vi "Write Humidifier T.vi"(8 "error in (no error)":errorcluster, 10 "Humidifier T":cluster{"Hum 1":sgl, "Hum 2":sgl}, 11 "cCRDS Data in":refnum<class "cCRDS Data.lvclass">=refnum) -> (0 "error out":errorcluster, 3 "cCRDS Data out":refnum<class "cCRDS Data.lvclass">)   [LabVIEW 2015, in "cCRDS Data.lvclass"]
uses:
  cCRDS Data.lvclass
  cCRDS Data.lvclass/cCRDS Data.ctl
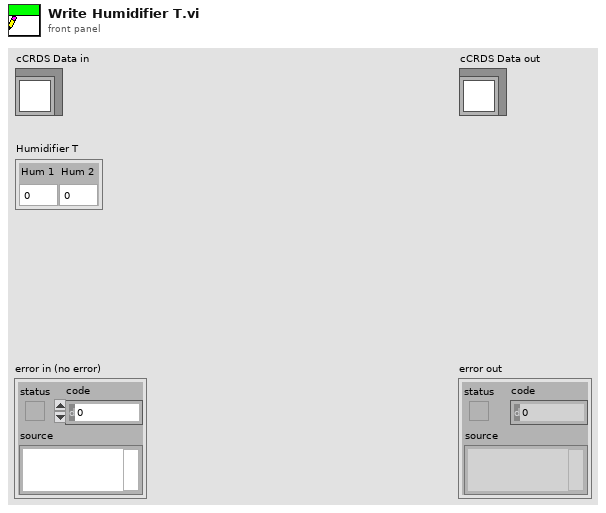
[diagram p1: front panel]
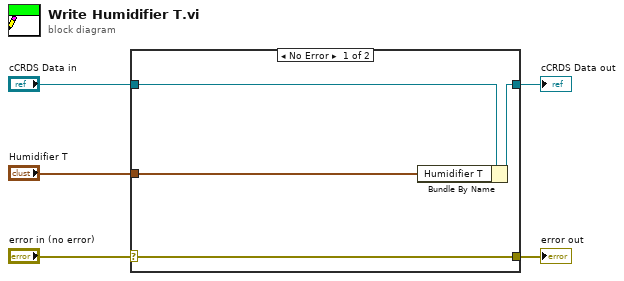
[diagram p0: block diagram]
diagram:
  n1 = case shown="No Error" "error in (no error)" {
    selector: "error in (no error)" -> [w9 w10]
    tunnel: [w9 w10] -> w4
    tunnel: [w7 w11] -> w2
    tunnel: "cCRDS Data in" -> [w8 w11]
    tunnel: "Humidifier T" -> [w6 _]
    frame No Error {
      n2 = Bundle By Name(cluster=w8, "Humidifier T"=w6) -> (w7:refnum<class "cCRDS Data.lvclass">)
    }
    frame Error {
    }
  }
  "error out" <- w4
  "cCRDS Data out" <- w2
